vi "Tear Down.vi"(8 "error in (no error)":errorcluster, 11 "User Interface in":refnum<class "User Interface.lvclass">) -> (0 "error out":errorcluster, 3 "User Interface out":refnum<class "User Interface.lvclass">)   [LabVIEW 2016, in "CLD Exam - ATM.lvlib" / "User Interface.lvclass"]
uses:
  User Interface.lvclass
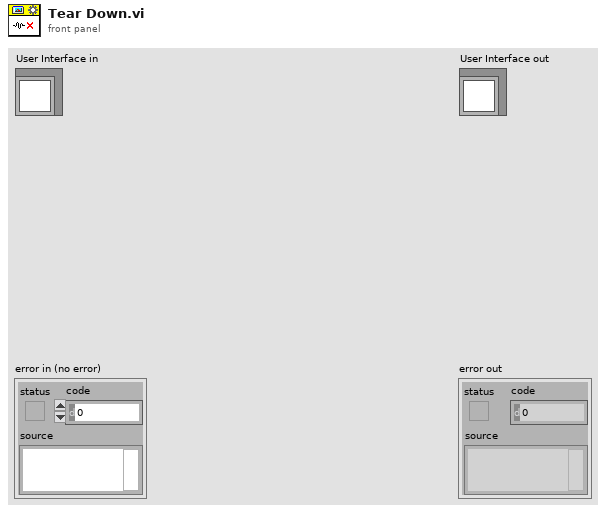
[diagram p1: front panel]
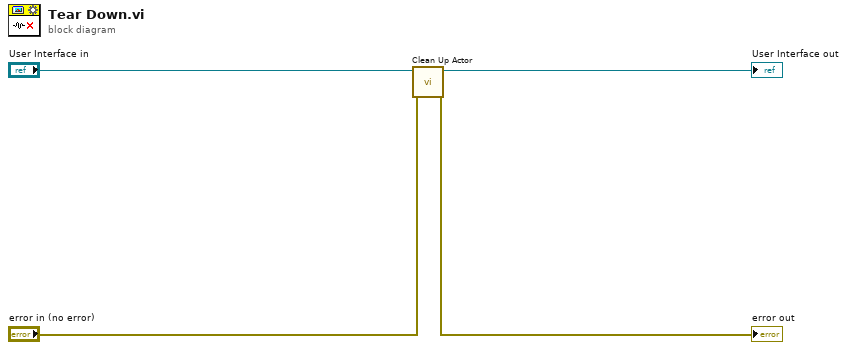
[diagram p0: block diagram]
diagram:
  n1 = call-dynamic "Clean Up Actor.vi"("error in (no error)"="error in (no error)", "User Interface in"="User Interface in") -> ("error out"=→"error out":errorcluster, "User Interface out"=→"User Interface out":refnum<class "User Interface.lvclass">)  [unwired: 8 in]
